vi "Read Row Parameters.vi"(8 "error in (no error)":errorcluster, 11 "id Manual":i32) -> (0 "error out":errorcluster, 1 "Total Acquisition Time":i32, 2 "DAQ Device Name":tag, 3 "Analog - Digital":bool, 4 "Digital Acquisition Parameters":T1 {"Execution Task Frequency" scale=1.0..100.0}, 5 "Analog Acquisition Parameters":T2={"sampling frequency Analog"=1000, "number of samples Analog"=1000, "Channels Analog"=[]} {"number of samples Analog" scale=0.0..2000.0; "sampling frequency Analog" scale=0.0..2000.0})   [LabVIEW 2020, in "Settings.lvlib"]
uses:
  Settings.lvlib
  Shared/AnalogAcquisitionParameters__typedef.ctl
  Shared/DigitalAcquisitionParameters__typedef.ctl
  <vilib>/drjdpowell/SQLite Library/SQL Connection/Open (path).vi
  <vilib>/drjdpowell/SQLite Library/SQL Connection/Open (string).vi
  <vilib>/AdvancedString/Path To Command Line String.vi
  <vilib>/drjdpowell/SQLite Library/SQL Connection/Execute SQL (1D String).vi
  <vilib>/drjdpowell/SQLite Library/SQL Connection/Connection.lvclass
  <vilib>/drjdpowell/SQLite Library/SQLite.lvlib
  Shared/Configuration for Acquisitions.lvlib
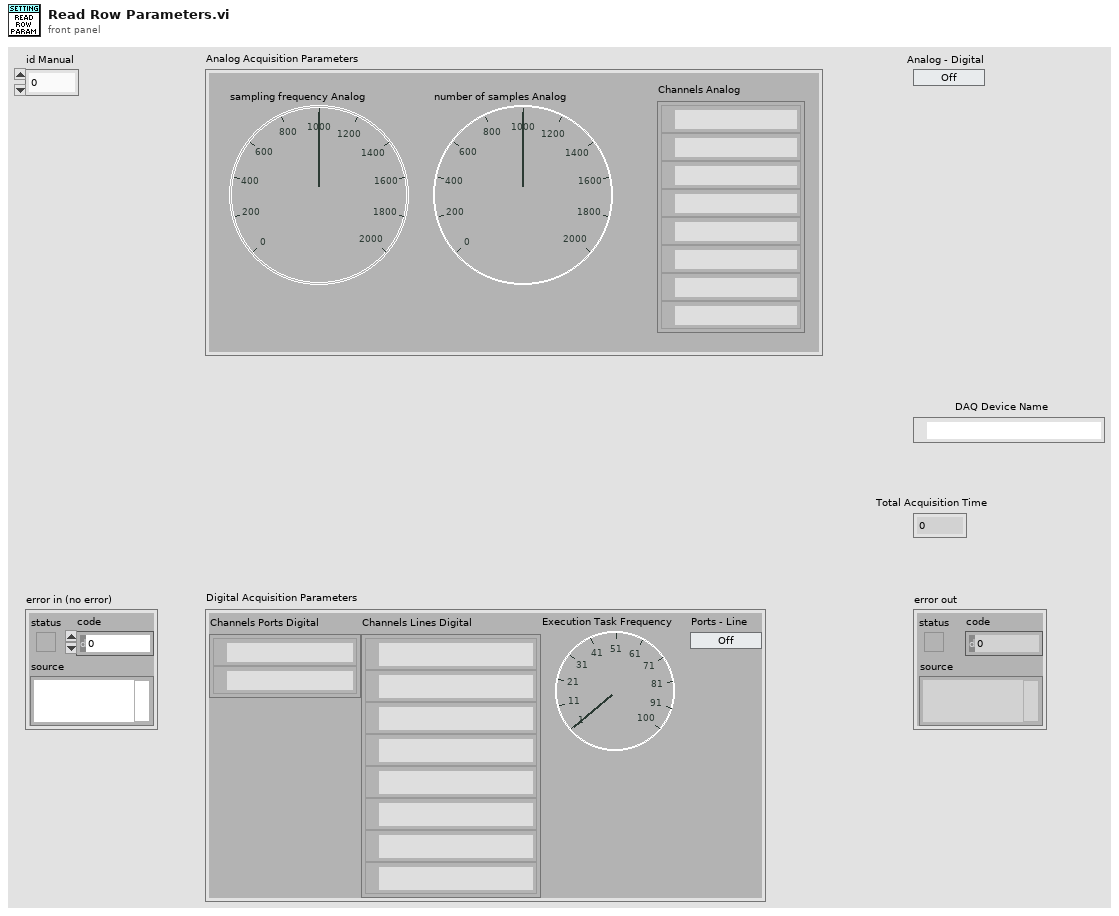
[diagram p1: front panel]
types:
  T1 = typedef "Configuration for Acquisitions.lvlib/DigitalAcquisitionParameters__typedef.ctl" = cluster{"Channels Ports Digital":tag[], "Channels Lines Digital":tag[], "Execution Task Frequency\n":u32, "Ports - Line":bool}
  T2 = typedef "Configuration for Acquisitions.lvlib/AnalogAcquisitionParameters__typedef.ctl" = cluster{"sampling frequency Analog":u32, "number of samples Analog":u32, "Channels Analog":tag[]}
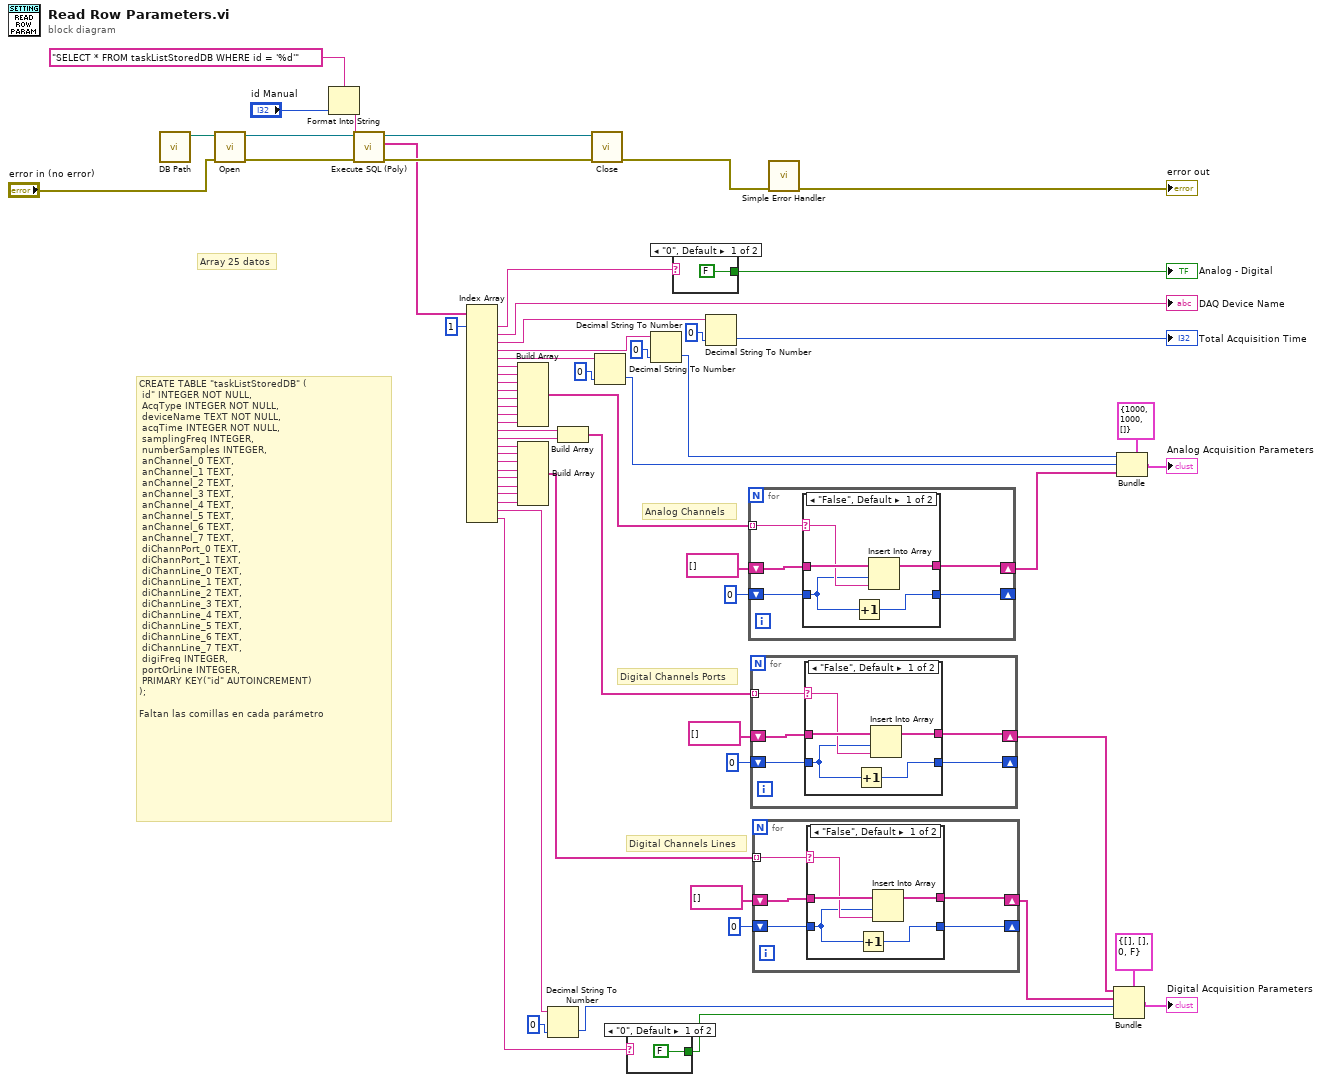
[diagram p0: block diagram]
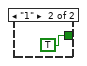
[diagram p5: hidden frame]
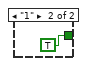
[diagram p6: hidden frame]
diagram:
  # "Digital Channels Lines"
  # "Digital Channels Ports"
  # "Analog Channels"
  # "CREATE TABLE \"taskListStoredDB\" (\n\tid\"\tINTEGER NOT NULL,\n\tAcqType\tINTEGER NOT NULL,\n\tdeviceName\tTEXT NOT NULL,\n\tacqTime\tINTEGER NOT NULL,\n\tsamplingFreq\tINTEGER,\n\tnumberSamples\tINTEGER,\n\tanChannel_0\tTEXT,\n\tanChannel_1\tTEXT,\n\tanChannel_2\tTEXT,\n\tanChannel_3\tTEXT,\n\tanChannel_4 TEXT,\n\tanChannel_5\tTEXT,\n\tanChannel_6\tTEXT,\n\tanChannel_7\tTEXT,\n\tdiChannPort_0\tTEXT,\n\tdiChannPort_1\tTEXT,\n\tdiChannLine_0\tTEXT,\n\tdiChannLine_1\tTEXT,\n\tdiChannLine_2\tTEXT,\n\tdiChannLine_3\tTEXT,\n\tdiChannLine_4\tTEXT,\n\tdiChannLine_5\tTEXT,\n\tdiChannLine_6\tTEXT,\n\tdiChannLine_7\tTEXT,\n\tdigiFreq\tINTEGER,\n\tportOrLine INTEGER,\n\tPRIMARY KEY(\"id\" AUTOINCREMENT)\n);\n\nFaltan las comillas en cada parámetro"
  # "Array 25 datos"
  n1 = call "DB Path.vi"() -> ("DB Path"=w58:path)  [unwired: 11 in]
  n2 = call-poly <vilib>:"Open.vi"("error in (no error)"="error in (no error)", "db file"=w58) -> ("error out"=w64:errorcluster, "SQLite Connection"=w61:refnum<class "Connection.lvclass">)  [unwired: 8 in]
  n3 = Format Into String(format string="SELECT * FROM taskListStoredDB WHERE id = '%d'" ("SQL"), "id Manual") -> (resulting string=w55:string)  [unwired: 2 in, 1 out]
  n4 = call-poly <vilib>:"Execute SQL (Poly).vi"("error in (no error)"=w64, "SQL"=w55, "SQLite Connection in"=w61) -> ("error out"=w62:errorcluster, "Result Set"=w52:string[], "SQLite Connection"=w60:refnum<class "Connection.lvclass">)  [unwired: 5 in, 1 out]
  n5 = Index Array(array=w52, index #1=1 ("index")) -> (element #1=w51:string, element #2=→"DAQ Device Name":string, element #3=w48:string, element #4=w43:string, element #5=w42:string, element #6=w38:string, element #7=w37:string, element #8=w36:string, element #9=w35:string, element #10=w34:string, element #11=w33:string, element #12=w32:string, element #13=w31:string, element #14=w29:string, element #15=w28:string, element #16=w25:string, element #17=w24:string, element #18=w23:string, element #19=w22:string, element #20=w21:string, element #21=w20:string, element #22=w19:string, element #23=w18:string, element #24=w16:string, element #25=w14:string)  [unwired: 24 in]
  n6 = Build Array(w38, w37, w36, w35, w34, w33, w32, w31) -> (w10:string[])
  n7 = Build Array(w25, w24, w23, w22, w21, w20, w19, w18) -> (w2:string[])
  n8 = Decimal String To Number(string=w16, default (0L)=0 ("default (0 I32)")) -> (number=w15:i32)  [unwired: 1 in, 1 out]
  n9 = Build Array(w29, w28) -> (w6:string[])
  n10 = call-dynamic "Close.vi"("error in (no error)"=w62, "SQLite Connection in"=w60) -> ("error out"=w57:errorcluster)  [unwired: 9 in]
  n11 = Decimal String To Number(string=w42, default (0L)=0 ("default (0 I32)")) -> (number=w39:i32)  [unwired: 1 in, 1 out]
  n12 = case shown="\"0\", Default" w14 {
    tunnel: [FALSE TRUE] -> w13
    frame "0", Default {
    }
    frame "1" {
    }
  }
  n13 = Decimal String To Number(string=w43, default (0L)=0 ("default (0 I32)")) -> (number=w40:i32)  [unwired: 1 in, 1 out]
  n14 = case shown="\"0\", Default" w51 {
    tunnel: [FALSE TRUE] -> w50
    frame "0", Default {
    }
    frame "1" {
    }
  }
  "Analog - Digital" <- w50
  n15 = Decimal String To Number(string=w48, default (0L)=0 ("default (0 I32)")) -> (number=→"Total Acquisition Time":i32)  [unwired: 1 in, 1 out]
  n16 = for {
    tunnel: w10 -> [w73] mode=indexing
    shift-right: [w71] -> w9
    shift-left: string[] [] -> [w72]
    shift-right: [w69] -> _
    shift-left: 0 -> [w70]
    n17 = case shown="\"False\", Default" w73 {
      selector: w73 -> [w77 _]
      tunnel: w72 -> [w78 w79]
      tunnel: [w76 w79] -> w71
      tunnel: w70 -> [w75 w80]
      tunnel: [w74 w80] -> w69
      frame "False", Default {
        n18 = Increment(x=w75) -> (x+1=w74:i32)
        n19 = Insert Into Array(array=w78, index=w75, new element=w77) -> (w76:string[])
      }
      frame "" {
      }
    }
  }
  n20 = for {
    tunnel: w6 -> [w85] mode=indexing
    shift-right: [w83] -> w5
    shift-left: string[] [] -> [w84]
    shift-right: [w81] -> _
    shift-left: 0 -> [w82]
    n21 = case shown="\"False\", Default" w85 {
      selector: w85 -> [w89 _]
      tunnel: w84 -> [w90 w91]
      tunnel: [w88 w91] -> w83
      tunnel: w82 -> [w87 w92]
      tunnel: [w86 w92] -> w81
      frame "False", Default {
        n22 = Increment(x=w87) -> (x+1=w86:i32)
        n23 = Insert Into Array(array=w90, index=w87, new element=w89) -> (w88:string[])
      }
      frame "" {
      }
    }
  }
  n24 = for {
    tunnel: w2 -> [w97] mode=indexing
    shift-right: [w95] -> w1
    shift-left: string[] [] -> [w96]
    shift-right: [w93] -> _
    shift-left: 0 -> [w94]
    n25 = case shown="\"False\", Default" w97 {
      selector: w97 -> [w101 _]
      tunnel: w96 -> [w102 w103]
      tunnel: [w100 w103] -> w95
      tunnel: w94 -> [w99 w104]
      tunnel: [w98 w104] -> w93
      frame "False", Default {
        n26 = Increment(x=w99) -> (x+1=w98:i32)
        n27 = Insert Into Array(array=w102, index=w99, new element=w101) -> (w100:string[])
      }
      frame "" {
      }
    }
  }
  n28 = call <vilib>:"Simple Error Handler.vi"("error in (no error)"=w57) -> ("error out"=→"error out":errorcluster)  [unwired: 4 in, 4 out]
  n29 = Bundle(cluster=T1 {"Channels Ports Digital"=[], "Channels Lines Digital"=[], "Execution Task Frequency\n"=0, "Ports - Line"=FALSE} ("Digital Acquisition Parameters"), "Channels Ports Digital"=w5, "Channels Lines Digital"=w1, "Execution Task Frequency"=w15, "Ports - Line"=w13) -> (→"Digital Acquisition Parameters":T1)
  n30 = Bundle(cluster=T2 {"sampling frequency Analog"=1000, "number of samples Analog"=1000, "Channels Analog"=[]} ("Analog Acquisition Parameters"), "sampling frequency Analog"=w40, "number of samples Analog"=w39, "Channels Analog"=w9) -> (→"Analog Acquisition Parameters":T2)
